vi "ConfigUtilities - Initialize Section Page Panel.vi"(7 "Packets Listbox":refnum<vi>, 8 "error in (no error)":errorcluster, 9 "Packet IDs Property":string, 10 "Packet Names Property":string, 11 "Item Ref in":T1 format="%.0x") -> (0 "error out":errorcluster, 1 "Channel IDs":i32[](array[numeric]), 2 "Channel Names":string[](array[string]), 3 "Item Ref out":T1 format="%.0x")   [LabVIEW 2015, in "UDP-Custom-Device System Explorer.lvlib"]
doc: "Initialize the Rx Channels Section Page Panel."
uses:
  UDP-Custom-Device System Explorer.lvlib
  <vilib>/NI Veristand/Custom Device API/Custom Device Item Ref.ctl
  <vilib>/Utility/miscctls.llb/LVRowAndColumnUnsignedTypeDef.ctl
  <vilib>/NI Veristand/Custom Device API/Get Item Property (String Array).vi
  <vilib>/NI Veristand/Custom Device API/Get Item Property (I32 Array).vi
  <vilib>/NI VeriStand/Custom Device API/Custom Device API.lvlib
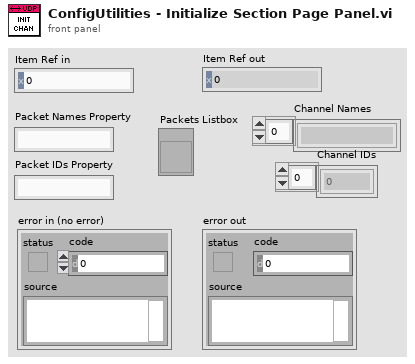
[diagram p1: front panel]
types:
  T1 = typedef "Custom Device API.lvlib/Custom Device Item Ref.ctl" = u64
  T2 = typedef "LVRowAndColumnUnsignedTypeDef.ctl" = cluster{"Row":u32, "Column":u32}
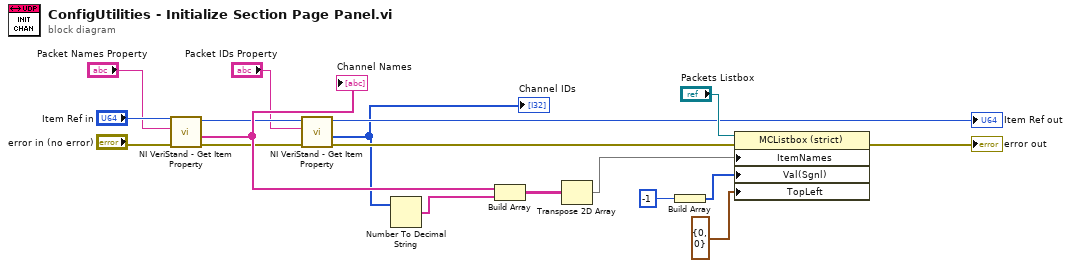
[diagram p0: block diagram]
diagram:
  n1 = call-poly <vilib>:"NI VeriStand - Get Item Property.vi"("error in (no error)"="error in (no error)", "Property Name"="Packet Names Property", "Item Ref in"="Item Ref in") -> ("error out"=w11:errorcluster, "Value"=w14:string[], "Item Ref out"=w10:T1)  [unwired: 5 in, 1 out]
  "Channel Names" <- w14
  n2 = call-poly <vilib>:"NI VeriStand - Get Item Property.vi"("error in (no error)"=w11, "Property Name"="Packet IDs Property", "Item Ref in"=w10) -> ("error out"=w15:errorcluster, "Value"=w2:i32[], "Item Ref out"=→"Item Ref out":T1)  [unwired: 5 in, 1 out]
  "Channel IDs" <- w2
  n3 = Number To Decimal String(number=w2) -> (decimal integer string=w1:string[])  [unwired: 1 in]
  n4 = Build Array(w14, w1) -> (w12:string[][])
  n5 = Transpose 2D Array(2D array=w12) -> (transposed array=w16:string[][])
  n6 = Build Array(-1) -> (w17:i32[])
  n7 = property class="MCListbox (strict)"(reference="Packets Listbox", error in=w15, "ItemNames"=w16, "Val(Sgnl)"=w17, "TopLeft"=T2 {"Row"=0, "Column"=0} ("Top Left Visible Cell")) -> (error out=→"error out":errorcluster)  [unwired: 1 out]
